vi "ramdomnumber.vi"() -> ()   [LabVIEW 2015]
panel:
  out "random (0 to 1)":dbl
  out "result":dbl
  out "Numeric":i32
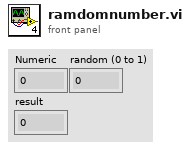
[diagram p1: front panel]
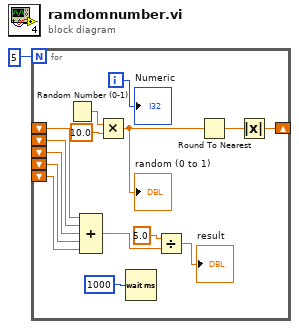
[diagram p0: block diagram]
diagram:
  n1 = for {
    N: 5 -> [_]
    shift-right: [w6] -> _
    shift-left: _ -> [w14]
    shift-left: _ -> [w13]
    shift-left: _ -> [w12]
    shift-left: _ -> [w11]
    shift-left: _ -> [w10]
    i -> [w15]
    n2 = Random Number (0-1)() -> (number: 0 to 1=w3:dbl)
    n3 = Compound Arithmetic op=ADD(w14, w13, w12, w11, w10) -> (w9:dbl)
    n4 = Multiply(x=w3, y=10.0) -> (x*y=w2:dbl)
    "random (0 to 1)" <- w2
    n5 = Wait (ms)(milliseconds to wait=u32 1000) -> ()  [unwired: 1 out]
    n6 = Divide(x=5.0, y=w9) -> (x/y=→"result":dbl)
    n7 = Round To Nearest(number=w2) -> (nearest integer value=w5:dbl)
    n8 = Absolute Value(x=w5) -> (abs(x)=w6:dbl)
    "Numeric" <- w15
  }
